vi "Read Data.vi"(8 "error in":errorcluster, 11 "CRDS Cell in":refnum<class "CRDS Cell.lvclass">) -> (0 "error out":errorcluster, 2 "CRDS Cell":refnum<class "CRDS Cell Data.lvclass">, 3 "CRDS Cell out":refnum<class "CRDS Cell.lvclass">)   [LabVIEW 2014, in "CRDS Lib.lvlib" / "CRDS Cell.lvclass"]
doc: "Retrieve the CRDS cell data."
uses:
  CRDS Cell.lvclass
  Data/Cell/CRDS Cell Data.lvclass
  CRDS Cell.lvclass/CRDS Cell.ctl
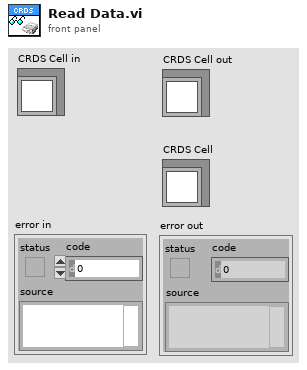
[diagram p1: front panel]
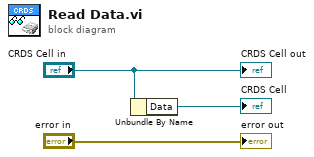
[diagram p0: block diagram]
diagram:
  n1 = Unbundle By Name("CRDS Cell in") -> ("Data"=→"CRDS Cell":refnum<class "CRDS Cell Data.lvclass">)
  "error out" <- "error in"
  "CRDS Cell out" <- "CRDS Cell in"
